vi "Find VIs by Pattern.vi"(8 "error in":errorcluster, 10 "pattern":string, 11 "Selction Owning Folder":path) -> (0 "error out":errorcluster, 2 "All Files in Dir":path[](array[path]))   [LabVIEW 2020, in "ConstantErrorsMaker.lvlib"]
uses:
  ConstantErrorsMaker.lvlib
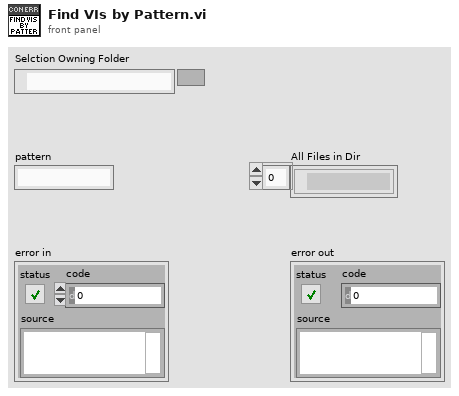
[diagram p1: front panel]
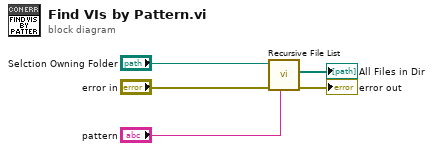
[diagram p0: block diagram]
diagram:
  n1 = call <vilib>:"Recursive File List.vi"("pattern"="pattern", "error in (no error)"="error in", "Folder Path"="Selction Owning Folder") -> ("error out"=→"error out":errorcluster, "All Files in Dir"=→"All Files in Dir":path[])  [unwired: 4 in, 3 out]
